vi "DSC_remove_bad_points.vi"(1 "Database Trace In":T1(array[cluster])) -> (0 "Database Trace Out":T1(array[cluster]))   [LabVIEW 2016]
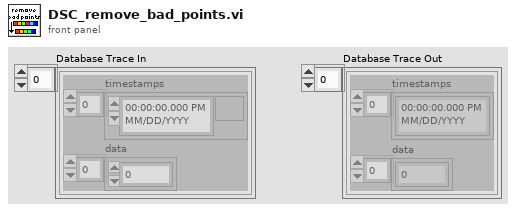
[diagram p1: front panel]
types:
  T1 = cluster{"timestamps":timestamp[], "data":dbl[]}[]
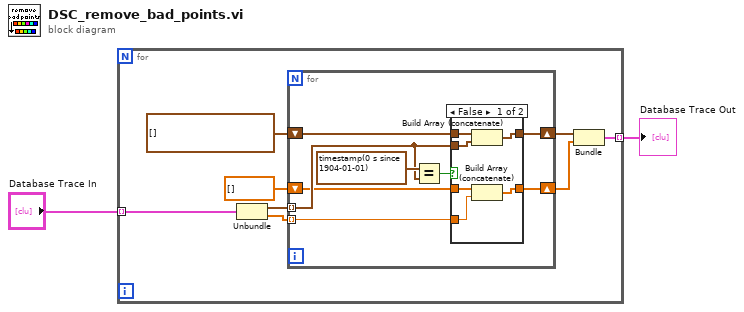
[diagram p0: block diagram]
diagram:
  n1 = for {
    tunnel: "Database Trace In" -> [w8] mode=indexing
    tunnel: [w3] -> w1 mode=indexing
    n2 = Unbundle(w8) -> ("timestamps"=w7:timestamp[], "data"=w6:dbl[])
    n3 = for {
      tunnel: w7 -> [w16] mode=indexing
      tunnel: w6 -> [w15] mode=indexing
      shift-right: [w14] -> w4
      shift-left: timestamp[] [] -> [w13]
      shift-right: [w12] -> w5
      shift-left: dbl[] [] -> [w11]
      n4 = Equal?(x=timestamp(0 s since 1904-01-01) ("Timestamp"), y=w16) -> (x = y?=w17:bool)
      n5 = case shown="False" w17 {
        tunnel: w16 -> [w24 _]
        tunnel: w15 -> [w21 _]
        tunnel: [w23 w25] -> w14
        tunnel: w13 -> [w22 w25]
        tunnel: [w20 w26] -> w12
        tunnel: w11 -> [w19 w26]
        frame False {
          n6 = Build Array (concatenate)(w22, w24) -> (w23:timestamp[])
          n7 = Build Array (concatenate)(w19, w21) -> (w20:dbl[])
        }
        frame True {
        }
      }
    }
    n8 = Bundle(w4, w5) -> (w3:cluster{timestamp[], dbl[]})  [unwired: 1 in]
  }
  "Database Trace Out" <- w1
